vi "PathPlanning.vi"() -> ()   [LabVIEW 2018]
uses:
  <vilib>/robotics/Navigation/shared/WorldMap/OccupancyGridWorldMap/NI_Robotics_OccupancyGridWorldMap.lvclass
  <vilib>/robotics/Navigation/NI_Robotics_Navigation .lvlib
  <vilib>/robotics/Obstacle Avoidance/Advanced Vector Field Histogram/NI_Robotics_Vector Field Histogram.lvlib
  <vilib>/Simulation/Implementation/XNodeFramework/SimXNode/SimX.xnode
  <vilib>/Simulation/Estimation/Implementation/NILVSim Discrete Kalman Filter.llb/SIM Disc KF Pred and Corr with Pred Gain with Checking Direct LV.vi
  C:/Program Files (x86)/National Instruments/LabVIEW 2018/vi.lib/robotics/Navigation/shared/WorldMap/AbstractDstarWorldMap/NI_Robotics_AbstractDstarWorldMap.lvclass
  C:/Program Files (x86)/National Instruments/LabVIEW 2018/vi.lib/robotics/Navigation/shared/WorldMap/AbstractWorldMap/NI_Robotics_AbstractWorldMap.lvclass
panel:
  in  "heading":T1
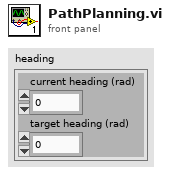
[diagram p1: front panel]
types:
  T1 = cluster{"current heading (rad)":dbl, "target heading (rad)":dbl}
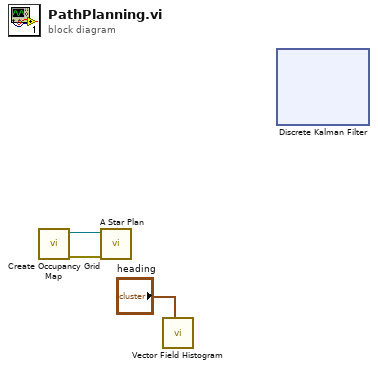
[diagram p0: block diagram]
diagram:
  n1 = call <vilib>:"Create Occupancy Grid Map.vi"() -> ("error out"=w2:errorcluster, "map reference out"=w3:refnum<data-value>, "occupancy grid"=w4:dbl[][])  [unwired: 9 in]
  n2 = call <vilib>:"A Star Plan.vi"("error in (no error)"=w2, "map reference in"=w3) -> ()  [unwired: 6 in, 4 out]
  n3 = call <vilib>:"Vector Field Histogram.vi"("heading"="heading") -> ()  [unwired: 7 in, 4 out]
  n4 = xnode "Discrete Kalman Filter"() -> ()  [unwired: 4 in, 8 out]
